vi "Get User VI Owners.vi"(8 "error in":errorcluster, 11 "User VI Ref":refnum<vi>) -> (0 "error out":errorcluster, 1 "Owner Filename (inc file extension)":string, 2 "Owner Path":path, 3 "User VI Owner Status":T1, 4 "Owner Filename (excluding file extension)":string, 5 "Owner Reference":refnum<vi>)   [LabVIEW 2021]
doc: "Gets details about the \"owners\" of the User VI. A VI could be owned by a library (.lvlib), a class (.lvclass) or a project (.lvproj)."
uses:
  Owner Status (enum).ctl
panel:
  # "Development\ncontrols/indicators useful for development and testing, but which are not outputs of the VI"
  # "Input\nInputs to the VI"
  # "Output\nOutputs of the VI"
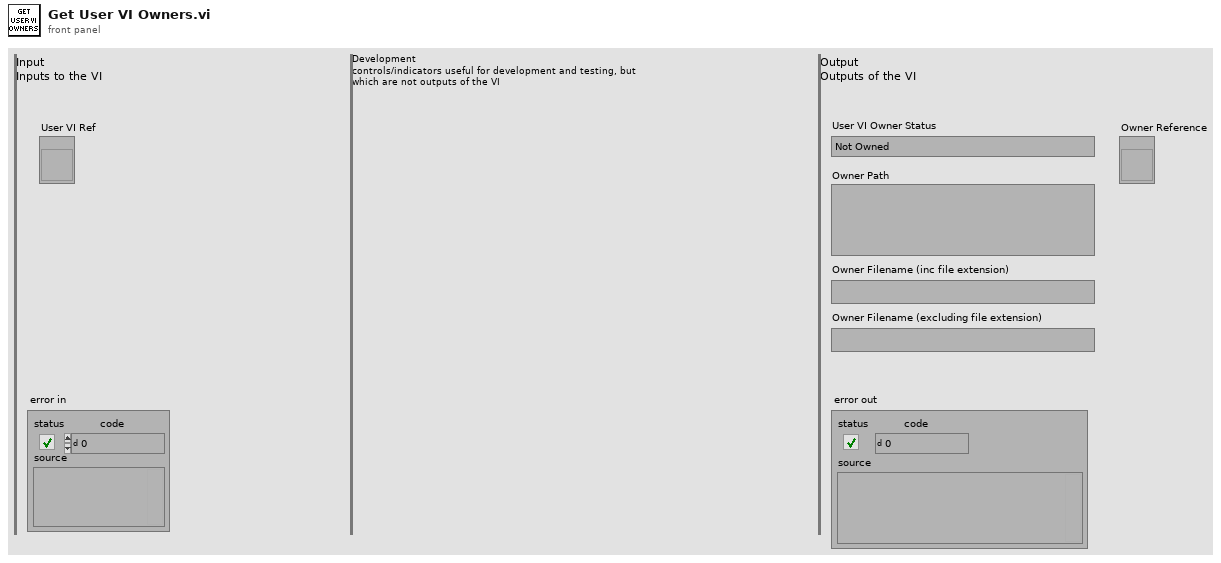
[diagram p1: front panel]
types:
  T1 = typedef "Owner Status (enum).ctl" = enum16{"Not Owned", "Owned by Library (lvlib)", "Owned by Class (lvclass)"}
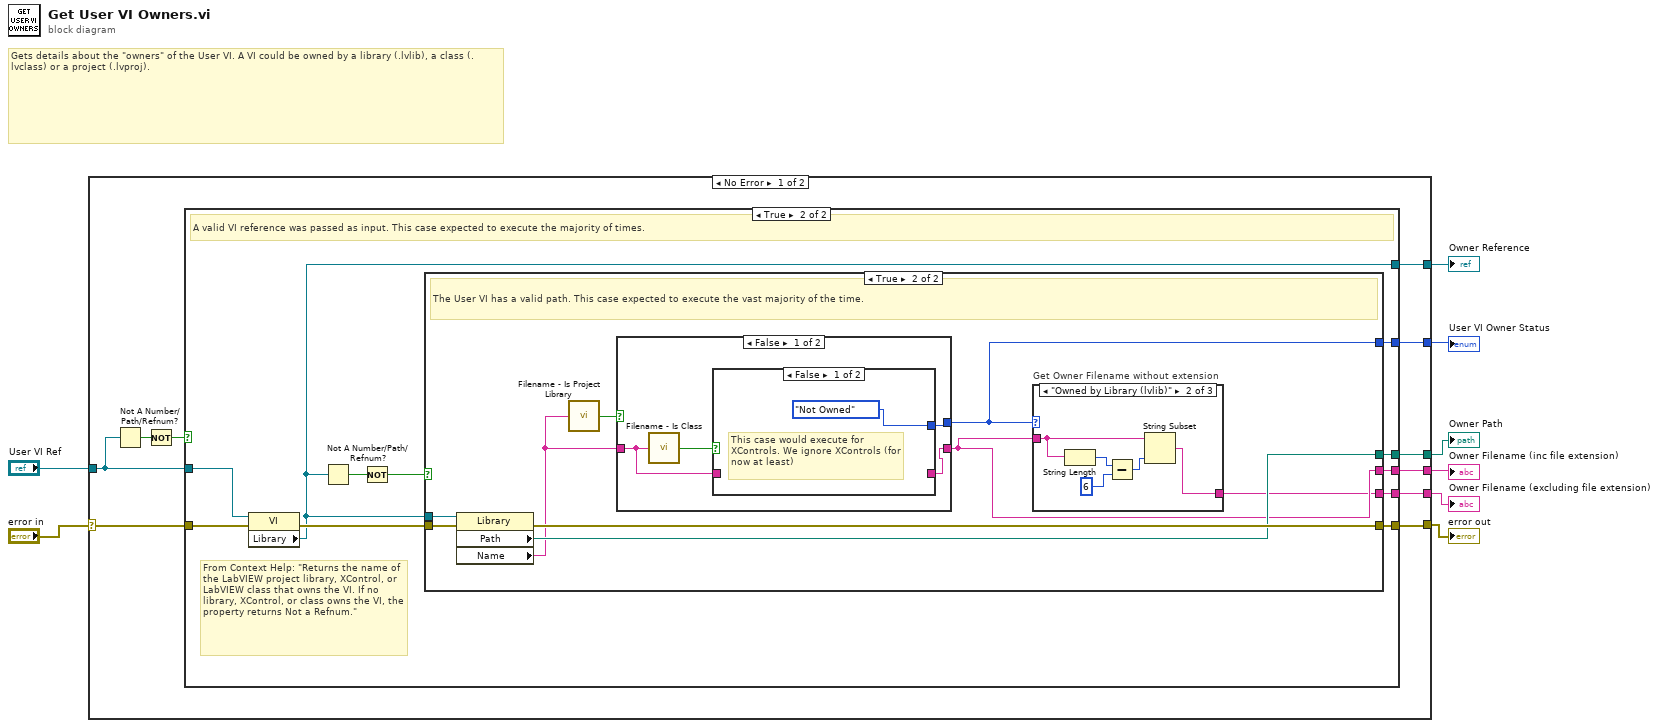
[diagram p0: block diagram]
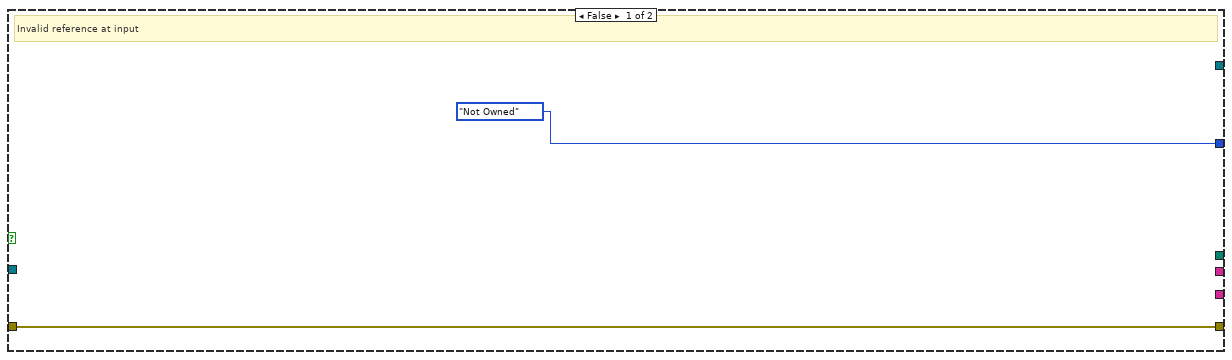
[diagram p2: hidden frame]
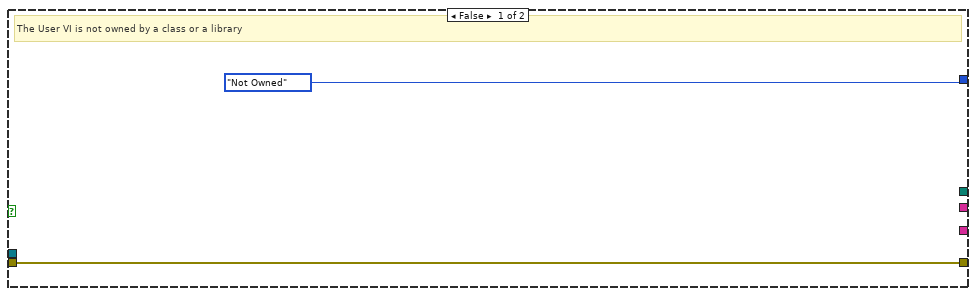
[diagram p3: hidden frame]
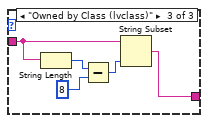
[diagram p5: hidden frame]
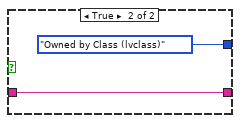
[diagram p6: hidden frame]
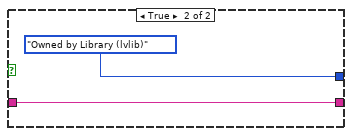
[diagram p7: hidden frame]
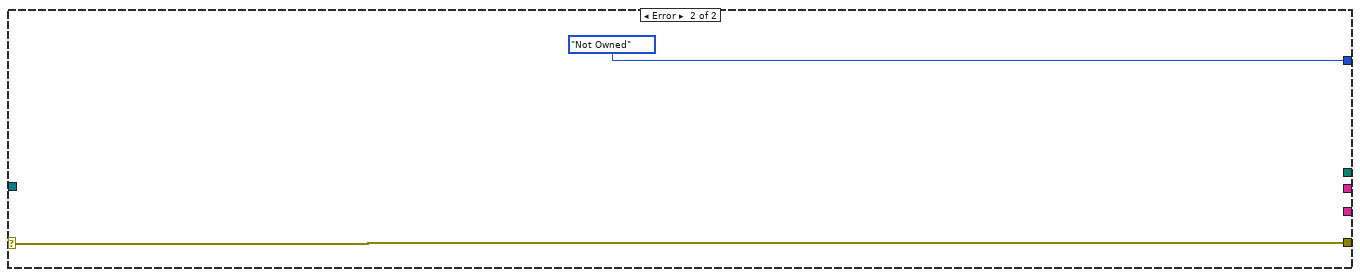
[diagram p8: hidden frame]
diagram:
  # "Gets details about the \"owners\" of the User VI. A VI could be owned by a library (.lvlib), a class (.lvclass) or a project (.lvproj)."
  n1 = case shown="No Error" "error in" {
    selector: "error in" -> [w18 w63]
    tunnel: [w17 w63] -> w7
    tunnel: "User VI Ref" -> [w16 _]
    tunnel: [w13 Owner_Status_(enum)."Not Owned" ("Owner Status")] -> w5
    tunnel: [w12 _] -> w4
    tunnel: [w11 _] -> w3
    tunnel: [w10 _] -> w2
    tunnel: [w9 _] -> w1
    frame No Error {
      n2 = Not A Number/Path/Refnum?(number/path/refnum=w16) -> (NaN/Path/Refnum?=w15:bool)
      n3 = Not(x=w15) -> (.not. x?=w14:bool)
      n4 = case shown="True" w14 {
        tunnel: w18 -> [w20 w31]
        tunnel: [w20 w25] -> w17
        tunnel: w16 -> [_ w28]
        tunnel: [Owner_Status_(enum)."Not Owned" ("Owner Status") w27] -> w13
        tunnel: [_ w24] -> w12
        tunnel: [_ w23] -> w11
        tunnel: [_ w22] -> w10
        tunnel: [_ w21] -> w9
        frame False {
          # "Invalid reference at input"
        }
        frame True {
          # "From Context Help: \"Returns the name of the LabVIEW project library, XControl, or LabVIEW class that owns the VI. If no library, XControl, or class owns the VI, the property returns Not a Refnum.\""
          # "A valid VI reference was passed as input. This case expected to execute the majority of times."
          n5 = property class="VI"(reference=w28, error in=w31) -> (error out=w26:errorcluster, "Library"=w21:refnum<vi>)  [unwired: 1 out]
          n6 = Not A Number/Path/Refnum?(number/path/refnum=w21) -> (NaN/Path/Refnum?=w30:bool)
          n7 = Not(x=w30) -> (.not. x?=w29:bool)
          n8 = case shown="True" w29 {
            tunnel: w21 -> [_ w41]
            tunnel: [Owner_Status_(enum)."Not Owned" ("Owner Status") w34] -> w27
            tunnel: w26 -> [w32 w42]
            tunnel: [w32 w40] -> w25
            tunnel: [_ w39] -> w24
            tunnel: [_ w36] -> w23
            tunnel: [_ w35] -> w22
            frame False {
              # "The User VI is not owned by a class or a library"
            }
            frame True {
              # "The User VI has a valid path. This case expected to execute the vast majority of the time."
              n9 = property class="Library"(reference=w41, error in=w42) -> (error out=w40:errorcluster, "Path"=w39:path, "Name"=w37:string)  [unwired: 1 out]
              n10 = call "Filename - Is Project Library.vi"("Filename (including file extension)"=w37) -> ("Is Project Library?"=w38:bool)
              n11 = case shown="False" w38 {
                tunnel: [w55 Owner_Status_(enum)."Owned by Library (lvlib)" ("Owner Status")] -> w34
                tunnel: w37 -> [w53 w60]
                tunnel: [w54 w60] -> w36
                frame False {
                  n12 = call "Filename - Is Class.vi"("Filename (including file extension)"=w53) -> ("Is Class?"=w56:bool)
                  n13 = case shown="False" w56 {
                    tunnel: [Owner_Status_(enum)."Not Owned" ("Owner Status") Owner_Status_(enum)."Owned by Class (lvclass)" ("Owner Status")] -> w55
                    tunnel: [_ w58] -> w54
                    tunnel: w53 -> [_ w58]
                    frame False {
                      # "This case would execute for XControls. We ignore XControls (for now at least)"
                    }
                    frame True {
                    }
                  }
                }
                frame True {
                }
              }
              n14 = case "Get Owner Filename without extension" shown="\"Owned by Library (lvlib)\"" w34 {
                tunnel: w36 -> [_ w47 w52]
                tunnel: [_ w43 w48] -> w35
                frame "Not Owned" {
                }
                frame "Owned by Library (lvlib)" {
                  n15 = String Length(string=w47) -> (length=w45:i32)
                  n16 = Subtract(x=w45, y=6) -> (x-y=w46:i32)
                  n17 = String Subset(string=w47, length (rest)=w46) -> (substring=w43:string)  [unwired: 1 in]
                }
                frame "Owned by Class (lvclass)" {
                  n18 = String Length(string=w52) -> (length=w50:i32)
                  n19 = Subtract(x=w50, y=8) -> (x-y=w51:i32)
                  n20 = String Subset(string=w52, length (rest)=w51) -> (substring=w48:string)  [unwired: 1 in]
                }
              }
            }
          }
        }
      }
    }
    frame Error {
    }
  }
  "error out" <- w7
  "User VI Owner Status" <- w5
  "Owner Filename (inc file extension)" <- w3
  "Owner Path" <- w4
  "Owner Filename (excluding file extension)" <- w2
  "Owner Reference" <- w1
